vi "StateCase.vi"(8 "Same State?":bool, 9 "StateIn":string, 10 "OutputsIn":T1, 11 "Inputs":T2) -> (2 "StateOut":string, 3 "OutputsOut":T1)   [LabVIEW 2014]
uses:
  state.lvsc/Outputs.ctl
  Stimulus.lvclass
  state.lvsc/Inputs.ctl
  Acquisition.lvclass
  Juicer.lvclass
  state.lvsc
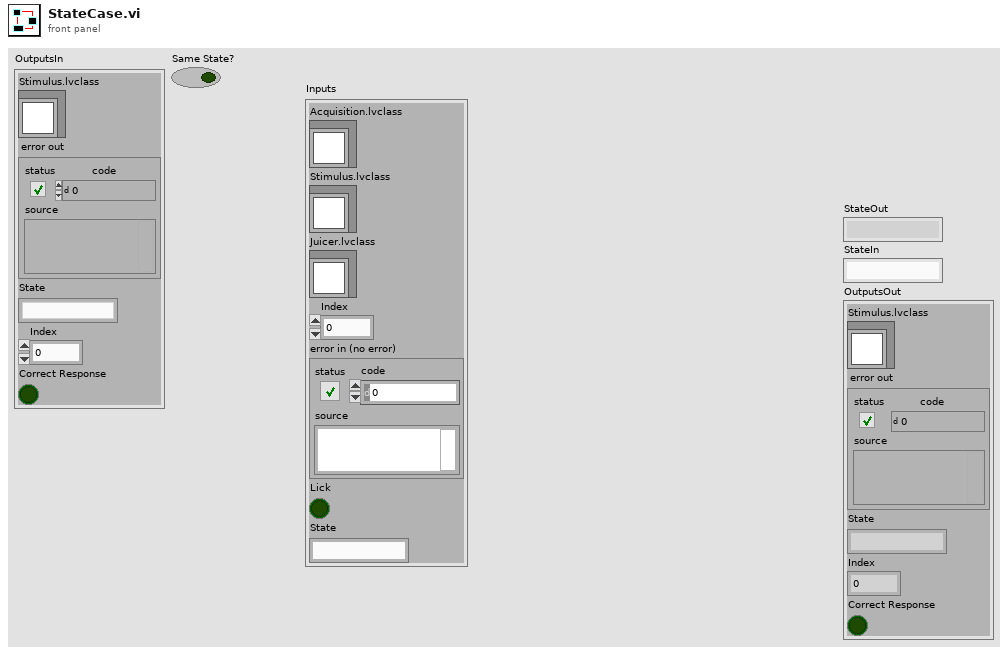
[diagram p1: front panel]
types:
  T1 = typedef "state.lvsc/Outputs.ctl" = cluster{"Stimulus.lvclass":refnum<class "Stimulus.lvclass">, "error out":errorcluster, "State":string, "Index":dbl, "Correct Response":bool}
  T2 = typedef "state.lvsc/Inputs.ctl" = cluster{"Acquisition.lvclass":refnum<class "Acquisition.lvclass">, "Stimulus.lvclass":refnum<class "Stimulus.lvclass">, "Juicer.lvclass":refnum<class "Juicer.lvclass">, "Index":dbl, "error in (no error)":errorcluster, "Lick":bool, "State":string}
  T3 = enum16{"Get Time", "Get Elapsed Time", "Reset Elapsed Time"}
  T4 = enum16{"air_delivery", "beh_session", "stim_periods", "licks", "liquid_delivery", ""}
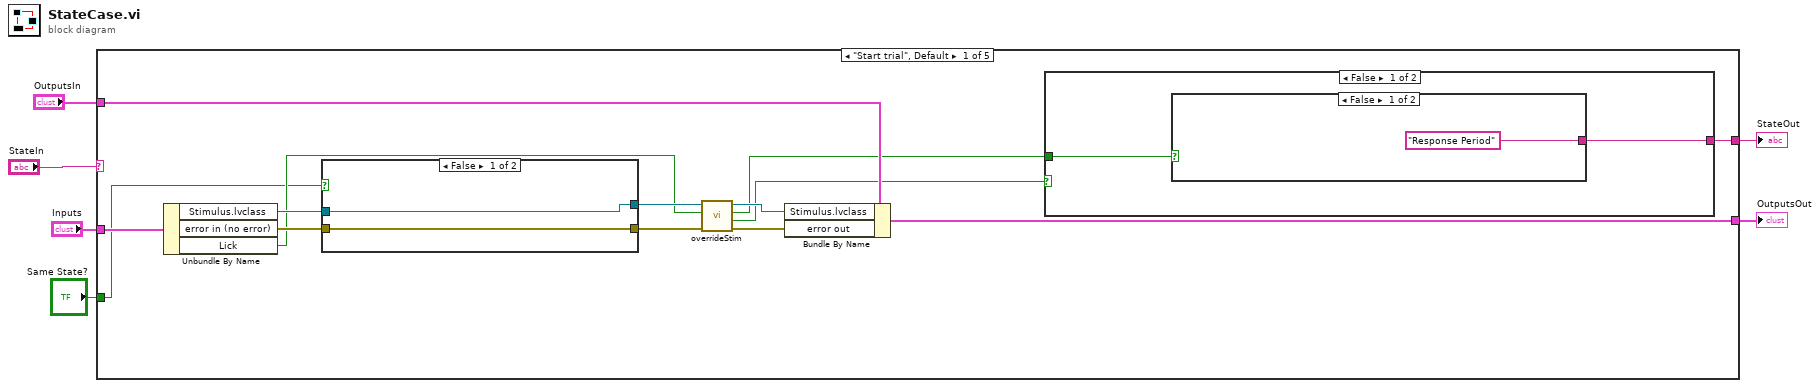
[diagram p0: block diagram]
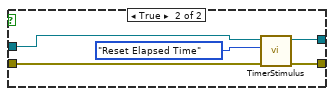
[diagram p2: hidden frame]
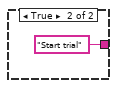
[diagram p3: hidden frame]
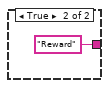
[diagram p4: hidden frame]
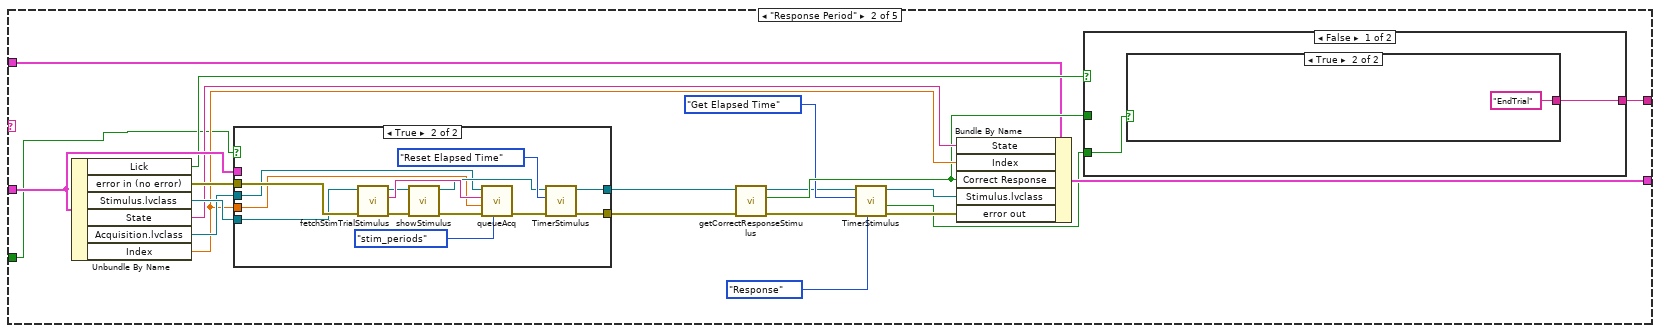
[diagram p5: hidden frame]
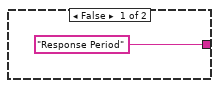
[diagram p7: hidden frame]
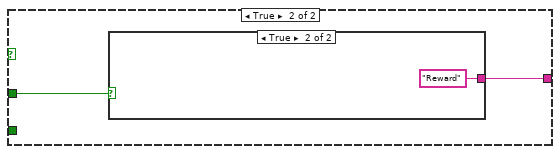
[diagram p8: hidden frame]
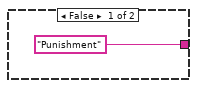
[diagram p9: hidden frame]
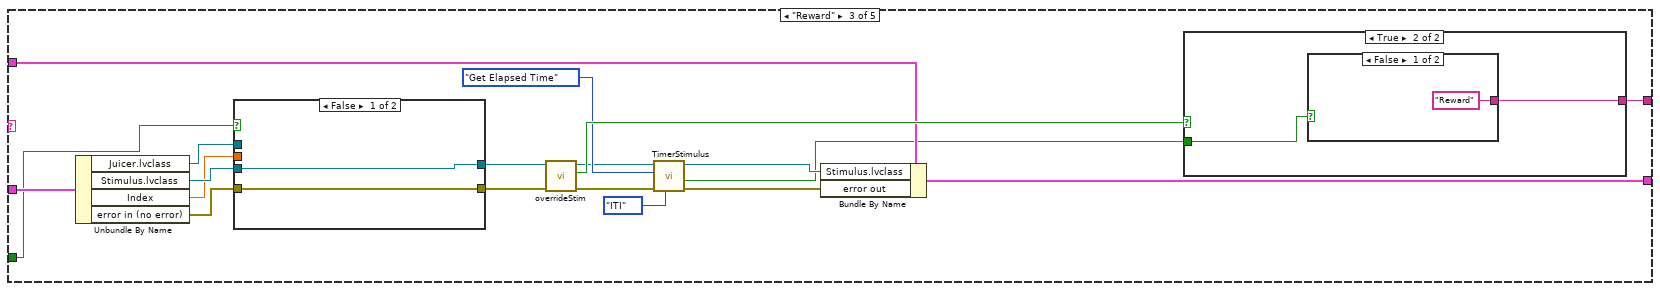
[diagram p10: hidden frame]
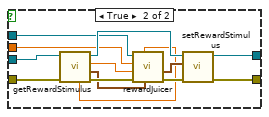
[diagram p11: hidden frame]
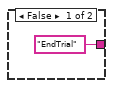
[diagram p12: hidden frame]
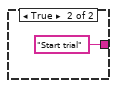
[diagram p13: hidden frame]
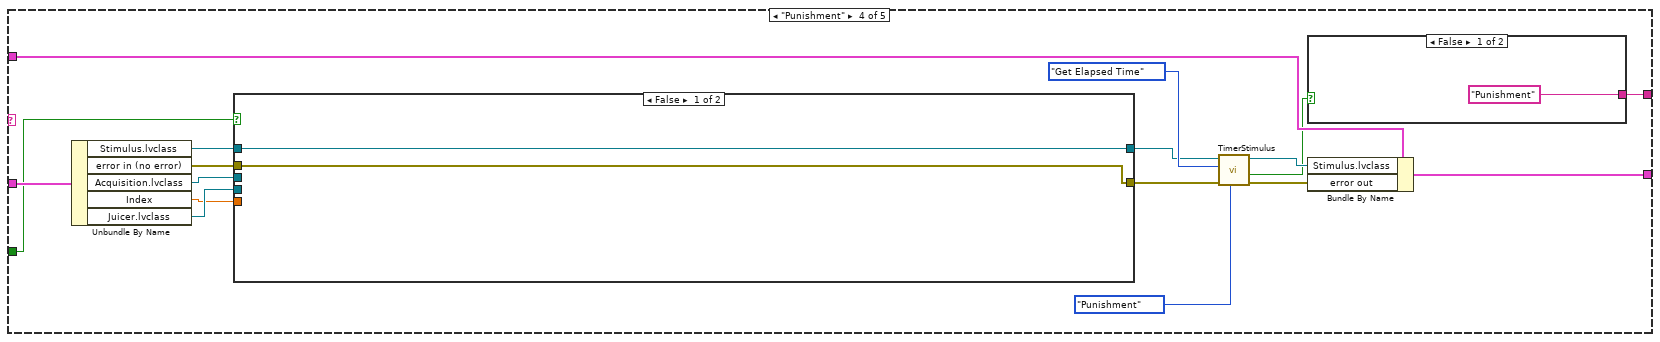
[diagram p14: hidden frame]
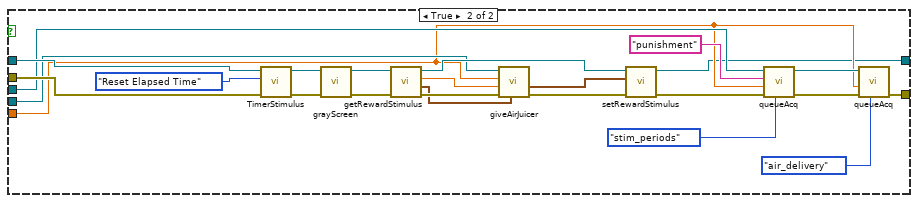
[diagram p15: hidden frame]
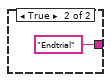
[diagram p16: hidden frame]
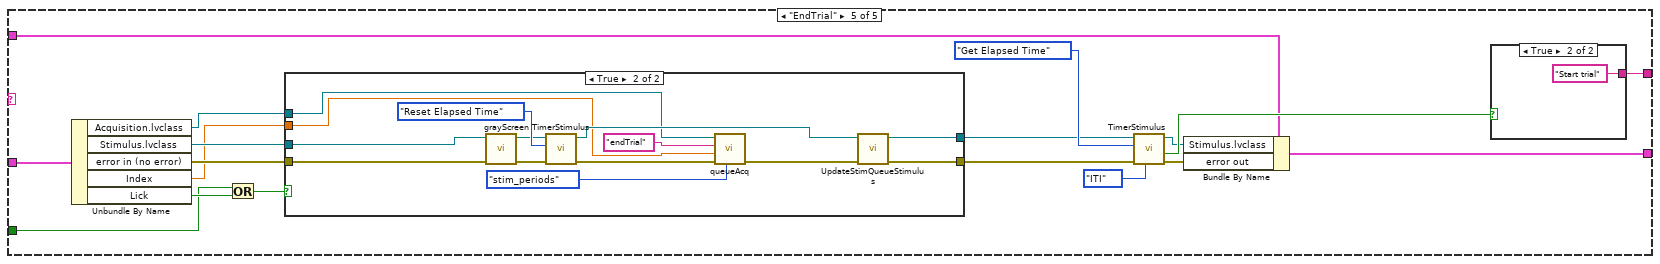
[diagram p17: hidden frame]
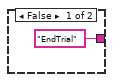
[diagram p19: hidden frame]
diagram:
  n1 = case shown="\"Start trial\", Default" "StateIn" {
    tunnel: [w20 w53 w96 w133 w179] -> w6
    tunnel: "Inputs" -> [w15 w52 w94 w132 w173]
    tunnel: [w16 w42 w79 w125 w172] -> w4
    tunnel: "OutputsIn" -> [w17 w41 w93 w131 w174]
    tunnel: "Same State?" -> [w7 w33 w78 w117 w162]
    frame "Start trial", Default {
      n2 = Unbundle By Name(w15) -> ("Stimulus.lvclass"=w19:refnum<class "Stimulus.lvclass">, "error in (no error)"=w18:errorcluster, "Lick"=w10:bool)
      n3 = case shown="False" w7 {
        tunnel: w19 -> [w22 w26]
        tunnel: [w22 w25] -> w14
        tunnel: [w21 w24] -> w13
        tunnel: w18 -> [w21 w23]
        frame False {
        }
        frame True {
          n4 = call-dynamic "TimerStimulus.vi"("error in (no error)"=w23, "Method"=T3."Reset Elapsed Time", "Stimulus in"=w26) -> ("error out"=w24:errorcluster, "Stimulus out"=w25:refnum<class "Stimulus.lvclass">)  [unwired: 5 in, 2 out]
        }
      }
      n5 = call-dynamic "overrideStim.vi"("error in (no error)"=w13, "Lick"=w10, "Stimulus in"=w14) -> ("error out"=w12:errorcluster, "Lick Override"=w9:bool, "Override"=w8:bool, "Stimulus out"=w11:refnum<class "Stimulus.lvclass">)  [unwired: 5 in]
      n6 = Bundle By Name(cluster=w17, "Stimulus.lvclass"=w11, "error out"=w12) -> (w16:T1)
      n7 = case shown="False" w9 {
        tunnel: [w29 "Reward"] -> w20
        tunnel: w8 -> [w28 _]
        frame False {
          n8 = case shown="False" w28 {
            tunnel: ["Response Period" "Start trial"] -> w29
            frame False {
            }
            frame True {
            }
          }
        }
        frame True {
        }
      }
    }
    frame "Response Period" {
      n9 = Unbundle By Name(w52) -> ("Lick"=w51:bool, "error in (no error)"=w50:errorcluster, "Stimulus.lvclass"=w49:refnum<class "Stimulus.lvclass">, "State"=w48:string, "Acquisition.lvclass"=w47:refnum<class "Acquisition.lvclass">, "Index"=w46:dbl)
      n10 = case shown="True" w33 {
        tunnel: w52 -> [_ _]
        tunnel: [w55 w56] -> w44
        tunnel: w50 -> [w55 w61]
        tunnel: w49 -> [w54 w60]
        tunnel: w47 -> [_ w59]
        tunnel: w46 -> [_ w58]
        tunnel: [w54 w57] -> w43
        frame False {
        }
        frame True {
          n11 = call-dynamic "fetchStimTrialStimulus.vi"("error in (no error)"=w61, "Stimulus in"=w60) -> ("error out"=w63:errorcluster, "Stim"=w68:string, "Stimulus out"=w62:refnum<class "Stimulus.lvclass">)  [unwired: 7 in]
          n12 = call-dynamic "showStimulus.vi"("error in (no error)"=w63, "Stimulus in"=w62) -> ("error out"=w67:errorcluster, "Stimulus out"=w65:refnum<class "Stimulus.lvclass">)  [unwired: 8 in]
          n13 = call-dynamic "queueAcq.vi"("table"=T4."stim_periods", "error in (no error)"=w67, "Window Number (0...15)"=w58, "period_type"=w68, "Acquisition in"=w59) -> ("error out"=w64:errorcluster)  [unwired: 4 in, 2 out]
          n14 = call-dynamic "TimerStimulus.vi"("error in (no error)"=w64, "Method"=T3."Reset Elapsed Time", "Stimulus in"=w65) -> ("error out"=w56:errorcluster, "Stimulus out"=w57:refnum<class "Stimulus.lvclass">)  [unwired: 5 in, 2 out]
        }
      }
      n15 = call-dynamic "getCorrectResponseStimulus.vi"("error in (no error)"=w44, "Stimulus in"=w43) -> ("error out"=w37:errorcluster, "Correct response"=w45:bool, "Stimulus out"=w38:refnum<class "Stimulus.lvclass">)  [unwired: 7 in]
      n16 = call-dynamic "TimerStimulus.vi"("Enum"=enum16{"Punishment", "ITI", "Response"}."Response", "error in (no error)"=w37, "Method"=T3."Get Elapsed Time", "Stimulus in"=w38) -> ("error out"=w36:errorcluster, "Timeout"=w34:bool, "Stimulus out"=w35:refnum<class "Stimulus.lvclass">)  [unwired: 4 in, 1 out]
      n17 = Bundle By Name(cluster=w41, "State"=w48, "Index"=w46, "Correct Response"=w45, "Stimulus.lvclass"=w35, "error out"=w36) -> (w42:T1)
      n18 = case shown="False" w51 {
        tunnel: [w71 w75] -> w53
        tunnel: w45 -> [_ w74]
        tunnel: w34 -> [w70 _]
        frame False {
          n19 = case shown="True" w70 {
            tunnel: ["Response Period" "EndTrial"] -> w71
            frame False {
            }
            frame True {
            }
          }
        }
        frame True {
          n20 = case shown="True" w74 {
            tunnel: ["Punishment" "Reward"] -> w75
            frame False {
            }
            frame True {
            }
          }
        }
      }
    }
    frame "Reward" {
      n21 = Unbundle By Name(w94) -> ("Juicer.lvclass"=w92:refnum<class "Juicer.lvclass">, "Stimulus.lvclass"=w91:refnum<class "Stimulus.lvclass">, "Index"=w89:dbl, "error in (no error)"=w90:errorcluster)
      n22 = case shown="False" w78 {
        tunnel: w92 -> [_ w104]
        tunnel: w91 -> [w98 w103]
        tunnel: w90 -> [w97 w102]
        tunnel: w89 -> [_ w101]
        tunnel: [w98 w100] -> w88
        tunnel: [w97 w99] -> w87
        frame False {
        }
        frame True {
          n23 = call-dynamic "getRewardStimulus.vi"("error in (no error)"=w102, "Stimulus in"=w103) -> ("error out"=w108:errorcluster, "Last Juice time"=w106:timestamp, "RI"=w105:dbl, "Stimulus out"=w109:refnum<class "Stimulus.lvclass">, "Pulse Duration"=w107:dbl)  [unwired: 5 in]
          n24 = call-dynamic "rewardJuicer.vi"("seconds since 1Jan1904 2"=w106, "pulse dur"=w107, "error in (no error)"=w108, "IRI"=w105, "Window Number (0...15)"=w101, "Juicer in"=w104) -> ("error out"=w111:errorcluster, "seconds since 1Jan1904"=w110:timestamp)  [unwired: 3 in, 1 out]
          n25 = call-dynamic "setRewardStimulus.vi"("error in (no error)"=w111, "Last Juice time"=w110, "Stimulus in"=w109) -> ("error out"=w99:errorcluster, "Stimulus out"=w100:refnum<class "Stimulus.lvclass">)  [unwired: 7 in]
        }
      }
      n26 = call-dynamic "overrideStim.vi"("error in (no error)"=w87, "Stimulus in"=w88) -> ("error out"=w83:errorcluster, "Override"=w95:bool, "Stimulus out"=w84:refnum<class "Stimulus.lvclass">)  [unwired: 6 in, 1 out]
      n27 = call-dynamic "TimerStimulus.vi"("Enum"=enum16{"Punishment", "ITI", "Response"}."ITI", "error in (no error)"=w83, "Method"=T3."Get Elapsed Time", "Stimulus in"=w84) -> ("error out"=w82:errorcluster, "Timeout"=w80:bool, "Stimulus out"=w81:refnum<class "Stimulus.lvclass">)  [unwired: 4 in, 1 out]
      n28 = Bundle By Name(cluster=w93, "Stimulus.lvclass"=w81, "error out"=w82) -> (w79:T1)
      n29 = case shown="True" w95 {
        tunnel: ["EndTrial" w114] -> w96
        tunnel: w80 -> [_ w113]
        frame False {
        }
        frame True {
          n30 = case shown="False" w113 {
            tunnel: ["Reward" "Start trial"] -> w114
            frame False {
            }
            frame True {
            }
          }
        }
      }
    }
    frame "Punishment" {
      n31 = Unbundle By Name(w132) -> ("Stimulus.lvclass"=w130:refnum<class "Stimulus.lvclass">, "error in (no error)"=w129:errorcluster, "Acquisition.lvclass"=w128:refnum<class "Acquisition.lvclass">, "Index"=w126:dbl, "Juicer.lvclass"=w127:refnum<class "Juicer.lvclass">)
      n32 = case shown="False" w117 {
        tunnel: w130 -> [w135 w142]
        tunnel: w129 -> [w134 w141]
        tunnel: w128 -> [_ w140]
        tunnel: w127 -> [_ w139]
        tunnel: w126 -> [_ w138]
        tunnel: [w134 w137] -> w121
        tunnel: [w135 w136] -> w122
        frame False {
        }
        frame True {
          n33 = call-dynamic "TimerStimulus.vi"("error in (no error)"=w141, "Method"=T3."Reset Elapsed Time", "Stimulus in"=w142) -> ("error out"=w154:errorcluster, "Stimulus out"=w151:refnum<class "Stimulus.lvclass">)  [unwired: 5 in, 2 out]
          n34 = call-dynamic "grayScreen.vi"("error in (no error)"=w154, "Stimulus in"=w151) -> ("error out"=w155:errorcluster, "Stimulus out"=w152:refnum<class "Stimulus.lvclass">)  [unwired: 8 in]
          n35 = call-dynamic "getRewardStimulus.vi"("error in (no error)"=w155, "Stimulus in"=w152) -> ("error out"=w156:errorcluster, "Last Juice time"=w147:timestamp, "RI"=w146:dbl, "Stimulus out"=w153:refnum<class "Stimulus.lvclass">)  [unwired: 5 in, 1 out]
          n36 = call-dynamic "giveAirJuicer.vi"("seconds since 1Jan1904 2"=w147, "error in (no error)"=w156, "IRI"=w146, "Window Number (0...15)"=w138, "Juicer in"=w139) -> ("error out"=w157:errorcluster, "seconds since 1Jan1904"=w159:timestamp)  [unwired: 4 in, 1 out]
          n37 = call-dynamic "setRewardStimulus.vi"("error in (no error)"=w157, "Last Juice time"=w159, "Stimulus in"=w153) -> ("error out"=w158:errorcluster, "Stimulus out"=w136:refnum<class "Stimulus.lvclass">)  [unwired: 7 in]
          n38 = call-dynamic "queueAcq.vi"("table"=T4."stim_periods", "error in (no error)"=w158, "Window Number (0...15)"=w138, "period_type"="punishment", "Acquisition in"=w140) -> ("error out"=w149:errorcluster, "Acquisition out"=w148:refnum<class "Acquisition.lvclass">)  [unwired: 4 in, 1 out]
          n39 = call-dynamic "queueAcq.vi"("table"=T4."air_delivery", "error in (no error)"=w149, "Window Number (0...15)"=w138, "Acquisition in"=w148) -> ("error out"=w137:errorcluster)  [unwired: 5 in, 2 out]
        }
      }
      n40 = call-dynamic "TimerStimulus.vi"("Enum"=enum16{"Punishment", "ITI", "Response"}."Punishment", "error in (no error)"=w121, "Method"=T3."Get Elapsed Time", "Stimulus in"=w122) -> ("error out"=w119:errorcluster, "Timeout"=w118:bool, "Stimulus out"=w120:refnum<class "Stimulus.lvclass">)  [unwired: 4 in, 1 out]
      n41 = case shown="False" w118 {
        tunnel: ["Punishment" "Endtrial"] -> w133
        frame False {
        }
        frame True {
        }
      }
      n42 = Bundle By Name(cluster=w131, "Stimulus.lvclass"=w120, "error out"=w119) -> (w125:T1)
    }
    frame "EndTrial" {
      n43 = Unbundle By Name(w173) -> ("Acquisition.lvclass"=w170:refnum<class "Acquisition.lvclass">, "Stimulus.lvclass"=w171:refnum<class "Stimulus.lvclass">, "error in (no error)"=w169:errorcluster, "Index"=w164:dbl, "Lick"=w163:bool)
      n44 = Or(x=w162, y=w163) -> (x .or. y?=w178:bool)
      n45 = case shown="True" w178 {
        tunnel: w171 -> [w181 w187]
        tunnel: w170 -> [_ w186]
        tunnel: w169 -> [w180 w185]
        tunnel: [w180 w184] -> w168
        tunnel: [w181 w183] -> w165
        tunnel: w164 -> [_ w182]
        frame False {
        }
        frame True {
          n46 = call-dynamic "grayScreen.vi"("error in (no error)"=w185, "Stimulus in"=w187) -> ("error out"=w190:errorcluster, "Stimulus out"=w188:refnum<class "Stimulus.lvclass">)  [unwired: 8 in]
          n47 = call-dynamic "TimerStimulus.vi"("error in (no error)"=w190, "Method"=T3."Reset Elapsed Time", "Stimulus in"=w188) -> ("error out"=w193:errorcluster, "Stimulus out"=w194:refnum<class "Stimulus.lvclass">)  [unwired: 5 in, 2 out]
          n48 = call-dynamic "queueAcq.vi"("table"=T4."stim_periods", "error in (no error)"=w193, "Window Number (0...15)"=w182, "period_type"="endTrial", "Acquisition in"=w186) -> ("error out"=w192:errorcluster)  [unwired: 4 in, 2 out]
          n49 = call-dynamic "UpdateStimQueueStimulus.vi"("error in (no error)"=w192, "Stimulus in"=w194) -> ("error out"=w184:errorcluster, "Stimulus out"=w183:refnum<class "Stimulus.lvclass">)  [unwired: 8 in]
        }
      }
      n50 = call-dynamic "TimerStimulus.vi"("Enum"=enum16{"Punishment", "ITI", "Response"}."ITI", "error in (no error)"=w168, "Method"=T3."Get Elapsed Time", "Stimulus in"=w165) -> ("error out"=w167:errorcluster, "Timeout"=w175:bool, "Stimulus out"=w166:refnum<class "Stimulus.lvclass">)  [unwired: 4 in, 1 out]
      n51 = Bundle By Name(cluster=w174, "Stimulus.lvclass"=w166, "error out"=w167) -> (w172:T1)
      n52 = case shown="True" w175 {
        tunnel: ["EndTrial" "Start trial"] -> w179
        frame False {
        }
        frame True {
        }
      }
    }
  }
  "StateOut" <- w6
  "OutputsOut" <- w4
